vi "HELGA_ECD.vi"() -> ()   [LabVIEW 2017]
panel:
  out "Methoden":T1(array[cluster])
  in  "Tab Control":T2(tab)
  in  "Dateiordner Housekeeping":path=path "C:/Users/Atmos/Desktop/Johnny"
  in  "Dateiname Housekeeping":string
  in  "DateiordnerECD1":path
  in  "DateinameECD1":string
  in  "DateiordnerECD2":path
  in  "DateinameECD2":string
  in  "Modul1/AI sicherer Bereich":dbl[][](array[numeric])=[[0.0, 0.0, 0.0, 0.0, 0.0, 0.0, 0.0, 0.0, 0.0, 0.0, 0.0, 0.0, 0.0, 0.0, 0.0, 0.0, 0.0, 0.0, 0.0, 0.0, 0.0, 0.0, 0.0, 0.0, 0.0, 0.0, 0.0, 0.0, 0.0, 0.0, 0.0, 0.0]]
  in  "Modul1/AIsNamen":string[](array[string])
  in  "Modul1/AI koeff":dbl[][](array[numeric])=[[0.0, 0.0, 0.0, 0.0, 0.0, 0.0, 0.0, 0.0, 0.0, 0.0, 0.0, 0.0, 0.0, 0.0, 0.0, 0.0, 0.0, 0.0, 0.0, 0.0, 0.0, 0.0, 0.0, 0.0, 0.0, 0.0, 0.0, 0.0, 0.0, 0.0, 0.0, 0.0]]
  in  "AIsNamenZurücksetzen":bool
  in  "Modul2/AIsNamen":string[](array[string])
  in  "Modul2/AI koeff":dbl[][](array[numeric])=[[0.0, 0.0, 0.0, 0.0, 0.0, 0.0, 0.0, 0.0, 0.0, 0.0, 0.0, 0.0, 0.0, 0.0, 0.0, 0.0, 0.0, 0.0, 0.0, 0.0, 0.0, 0.0, 0.0, 0.0, 0.0, 0.0, 0.0, 0.0, 0.0, 0.0, 0.0, 0.0]]
  in  "Modul2/AI sicherer Bereich":dbl[][](array[numeric])=[[0.0, 0.0, 0.0, 0.0, 0.0, 0.0, 0.0, 0.0, 0.0, 0.0, 0.0, 0.0, 0.0, 0.0, 0.0, 0.0, 0.0, 0.0, 0.0, 0.0, 0.0, 0.0, 0.0, 0.0, 0.0, 0.0, 0.0, 0.0, 0.0, 0.0, 0.0, 0.0]]
  in  "Modul3/AIsNamen":string[](array[string])
  in  "Modul3/AI koeff":dbl[][](array[numeric])=[[0.0, 0.0, 0.0, 0.0, 0.0, 0.0, 0.0, 0.0, 0.0, 0.0, 0.0, 0.0, 0.0, 0.0, 0.0, 0.0, 0.0, 0.0, 0.0, 0.0, 0.0, 0.0, 0.0, 0.0, 0.0, 0.0, 0.0, 0.0, 0.0, 0.0, 0.0, 0.0]]
  in  "Modul3/AI sicherer Bereich":dbl[][](array[numeric])=[[0.0, 0.0, 0.0, 0.0, 0.0, 0.0, 0.0, 0.0, 0.0, 0.0, 0.0, 0.0, 0.0, 0.0, 0.0, 0.0, 0.0, 0.0, 0.0, 0.0, 0.0, 0.0, 0.0, 0.0, 0.0, 0.0, 0.0, 0.0, 0.0, 0.0, 0.0, 0.0]]
  in  "Traps/MachsKoeff R(U)":dbl[][](array[numeric])=[[0.0, 0.0, 0.0, 0.0, 0.0, 0.0, 0.0, 0.0, 0.0, 0.0, 0.0, 0.0, 0.0, 0.0, 0.0, 0.0, 0.0, 0.0, 0.0, 0.0, 0.0, 0.0, 0.0, 0.0, 0.0, 0.0, 0.0, 0.0, 0.0, 0.0, 0.0, 0.0]]
  out "Schnelle Heizungen":string[](array[string])
  in  "Traps/MachsKoeff T(R)":dbl[][](array[numeric])=[[0.0, 0.0, 0.0, 0.0, 0.0, 0.0, 0.0, 0.0, 0.0, 0.0, 0.0, 0.0, 0.0, 0.0, 0.0, 0.0, 0.0, 0.0, 0.0, 0.0, 0.0, 0.0, 0.0, 0.0, 0.0, 0.0, 0.0, 0.0, 0.0, 0.0, 0.0, 0.0]]
  in  "Traps/Machs sicherer Bereich":dbl[][](array[numeric])=[[0.0, 0.0, 0.0, 0.0, 0.0, 0.0, 0.0, 0.0, 0.0, 0.0, 0.0, 0.0, 0.0, 0.0, 0.0, 0.0, 0.0, 0.0, 0.0, 0.0, 0.0, 0.0, 0.0, 0.0, 0.0, 0.0, 0.0, 0.0, 0.0, 0.0, 0.0, 0.0]]
  in  "LangsameHeizungen":string[](array[string])
  in  "ModuleLH":i32[](array[numeric]) min=1 max=3 step=1
  in  "AIsLH":i32[](array[numeric]) min=0 max=31 step=1
  in  "LHGruppe":bool[](array[boolean])
  in  "DIOsMod0Name":string[](array[string])
  in  "DIOsMod0Nr":i32[](array[numeric]) min=0 max=63 step=1
  in  "DIOsMod1Name":string[](array[string])
  in  "DIOsMod1Nr":i32[](array[numeric]) min=0 max=63 step=1
  in  "DIOsMod2AName":string[](array[string])
  in  "DIOsMod2ANr":i32[](array[numeric]) min=0 max=63 step=1
  in  "DIOsMod2BName":string[](array[string])
  in  "DIOsMod2BNr":i32[](array[numeric]) min=0 max=63 step=1
  out "AnzahlRegler/Modul":i32[](array[numeric])
  in  "Regler für den Probenfluß":i32
  in  "ReglerNameMod0":string[](array[string])
  in  "ReglerNameMod1":string[](array[string])
  in  "ReglerNameMod2A":string[](array[string])
  in  "ReglerNameMod2B":string[](array[string])
  in  "MWabfragenMod0":string[](array[string])=[":060F0401210120", ":06100401210120", ":06110401210120"]
  in  "MWabfragenMod1":string[](array[string])=[":060F0401210120", ":06100401210120", ":06110401210120"]
  in  "MWabfragenMod2A":string[](array[string])=[":060F0401210120", ":06100401210120", ":06110401210120"]
  in  "MWabfragenMod2B":string[](array[string])=[":060F0401210120", ":06100401210120", ":06110401210120"]
  in  "SPvorgebenMod0":string[](array[string])=[":060F020121", ":0610020121", ":0611020121"]
  in  "SPvorgebenMod1":string[](array[string])=[":060F020121", ":0610020121", ":0611020121"]
  in  "SPvorgebenMod2A":string[](array[string])=[":060F020121", ":0610020121", ":0611020121"]
  in  "SPvorgebenMod2B":string[](array[string])=[":060F020121", ":0610020121", ":0611020121"]
  in  "FaktorMod0":dbl[](array[numeric])=[9.375e-05, 9.375e-05, 9.375e-05]
  in  "FaktorMod1":dbl[](array[numeric])=[9.375e-05, 9.375e-05, 9.375e-05]
  in  "FaktorMod2A":dbl[](array[numeric])=[9.375e-05, 9.375e-05, 9.375e-05]
  in  "FaktorMod2B":dbl[](array[numeric])=[9.375e-05, 9.375e-05, 9.375e-05]
  in  "MWAntwortMod0":string[](array[string])=[":060F020121", ":0610020121", ":0611020121"]
  in  "MWAntwortMod1":string[](array[string])=[":060F020121", ":0610020121", ":0611020121"]
  in  "MWAntwortMod2A":string[](array[string])=[":060F020121", ":0610020121", ":0611020121"]
  in  "MWAntwortMod2B":string[](array[string])=[":060F020121", ":0610020121", ":0611020121"]
  in  "ReglerMod0 sicherer Bereich":dbl[][](array[numeric])=[[9.375e-05, 9.375e-05, 9.375e-05]]
  in  "ReglerMod1 sicherer Bereich":dbl[][](array[numeric])=[[9.375e-05, 9.375e-05, 9.375e-05]]
  in  "ReglerMod2A sicherer Bereich":dbl[][](array[numeric])=[[9.375e-05, 9.375e-05, 9.375e-05]]
  in  "ReglerMod2B sicherer Bereich":dbl[][](array[numeric])=[[9.375e-05, 9.375e-05, 9.375e-05]]
  in  "Metavariablen grüner Bereich":dbl[][](array[numeric])=[[0.0, 0.0, 0.0, 0.0, 0.0, 0.0, 0.0, 0.0, 0.0, 0.0, 0.0, 0.0, 0.0, 0.0, 0.0, 0.0, 0.0, 0.0, 0.0, 0.0, 0.0, 0.0, 0.0, 0.0, 0.0, 0.0, 0.0, 0.0, 0.0, 0.0, 0.0, 0.0]]
  in  "Metavariablen":string[](array[string])
  in  "Startmethode":i32=1
  in  "MethodeLöschen":bool
  in  "MethodeDuplizieren":bool
  in  "T_MainMach2":dbl[](array[numeric])
  in  "t_MainMach2":dbl[](array[numeric])
  in  "T_MainMach1":dbl[](array[numeric])
  in  "t_MainMach1":dbl[](array[numeric])
  in  "EinstellungenSpeichern":bool
  out "LangsameHeizungen":string[](array[string])
  in  "AllesSpeichern":bool
  in  "Methodenname":string
  in  "Int.Stop2":dbl
  in  "Int.Start2":dbl
  in  "Int.Stop1":dbl
  in  "Int.Start1":dbl
  in  "ZeitpktMS-2":dbl
  in  "ZeitpktMS-1":dbl
  in  "SPMPV":i32[](array[numeric])
  in  "ZeitpunkteMPV":dbl[](array[numeric])
  in  "Wert2":dbl
  in  "Vergleichsoperator2":dbl(ring) items=["<", "<=", "=", ">=", ">", "=/="]
  in  "AbfragbareVariablen2":dbl(ring) items=["T1-Trap1 [°C]", "T1-Trap2 [°C]", "T1-StirlingKühlkopf [°C]", "T1-PreCol1 [°C]", "T1-PreCol2 [°C]", "T1-MainCol1a [°C]", "T1-MainCol1b [°C]", "T1-MainCol2a [°C]", "T1-MainCol2b [°C]", "T1-Bronkhorst1a [°C]", "T1-Bronkhorst1b [°C]", "T1-Bronkhorst2a [°C]", "T1-Bronkhorst2b [°C]", "T1-2Pos1B [°C]", "T1-Spare9", "T1-2Pos1A [°C]", "T1-Spare10", "T1-TurboPump [°C]", "T1-StirlingPlatine [°C]", "T1-Spare5", "T1-Spare6", "T1-Spare7", "T1-Spare8", "F1-MFM1", "F1-MFM0D [mL]", "P1-HeliumHP [bara]", "P1-HeliumLP [bara]", "P1-PumpVordruck [mbara]", "TurboSpeed", "I1-MS-AC [A]", "I1-Trap1 [A]", "I1-Trap2 [A]", "T2-ECD1a", "T2-ECD1b", "T2-ECD2a", "T2-ECD2b", "T2-Col1a", "T2-Col1b", "T2-Col2a", "T2-Col2b", "T2-Spare1", "T2-Spare2", "T2-Oven_a", "T2-Oven_b", "T2-Spare3", "T2-Spare4", "T2-Spare5", "F2-MFM0", "F2-MFM2A", "F2-MFM2B", "P2-N2O_HP", "P2-N2O_LP", "P2-CO2_HP", "P2-CO2_LP", "AI-Spare1", "FL-MFM1000mL", "AI-Spare3", "AI-Spare4", "StirlingAlarm", "StirlingEmerg.", "AI-Spare7", "AI-Spare8", "AI-Spare9", "FL-MFM30mL", "T0-DC/DC5", "I0-24V_M0", "I0-48V_M1", "I0-24V_M1", "I0-28V_M2", "T0-Spare3", "T0-Spare2", "T0-Spare4", "T0-DC/DC7", "I0-20V_Laptop", "I0-28V_M1", "I0-24V_M2", "I0-12V_Licor", "T0-Spare1", "T0-Drier", "T0-Spare5", "F0-MFM0A [L]", "TL-Licor_a", "P0-Span-HP", "P0-spare1", "P0-Stickstoff-LP", "P0-Helium-LP", "P0-Cal-HP", "P0-P9Tavco[bar]", "F0-MFM0B [L]", "TL-Licor_b", "P0-Span-LP", "P0-spare2", "P0-Stickstoff-HP", "P0-Helium-HP", "P0-Cal-LP", "F0-MFM3", "T-Trap1", "T-Trap2", "T-PreMach1", "T-PreMach2", "T-MainMach1", "T-MainMach2", "PrC0 [bara]", "PrC0-Licor [bara]", "PrC1-Säule1 [bara]", "PrC1-Säule2 [bara]", "MFC1-Sample [ml/min]", "PrC1-BackFlush1 [bara]", "PrC1-BackFlush2 [bara]", "MFC1-Reaktant [l/min]", "MFC2A[ml/min]", "MFC2B[ml/min]", "MFC2C[ul/min]", "PrC2A[bara]", "MFC2D[ml/min]", "MFC2E[ml/min]", "PrC2B[bara]", "Gesamte Zeit", "Methodenzeit", "Zykluszeit Mod0", "Zykluszeit Mod1", "Zykluszeit Mod2A", "Zykluszeit Mod2B", "PositionMPV", "OverflowB", "OverflowA", "StirlingAlarmAlarm!"]
  in  "Dateien fürs MS schicken?":bool
  in  "Zwangsbedingungen":dbl[][](array[numeric])
  out "ZwangsBedingungen":string[][](array[string])
  in  "löschen":bool
  in  "Bedingung Nr. X":i32
  in  "Bedingung übernehmen":bool
  in  "Ausgangswert":dbl
  in  "BedienbareVariablen":dbl(ring) items=["D0-48V_M1", "D0-28V_M1", "D0-Pump2", "DL-LiCalS1H", "D-Spare2", "D-Spare4", "D0-28V_M2", "D0-Pump1", "D0-S01/EV1", "DL-Licor", "D0-EV3", "D0-EV2", "D1-StopMS", "D1-StartMS", "D1-TrapEvac1", "D1-TrapEvac2", "D1-2Pos1A", "D1-2Pos1B", "D1-TurboPump", "D1-PrePump", "D1-VacPump1", "D1-VacPump2", "D1-Stirling", "D1-P_MS", "D1-S1B(7)", "D1-S1A(6)", "D1-S1G", "D1-Fan3", "D1-LüfterMach1", "D1-LüfterMach2", "D1-MS-Power", "D2-SpülflußA", "D2-2Pos2A", "D2-Probe2A", "D2-ECD1HeaterOff", "D2-Fan1", "D2-Fan2", "D2-Spülfluß2B", "D2-2Pos2B", "D2-Probe2B", "D2-ECD2HeaterOff", "Heizen?Trap1", "Heizen?Trap2", "Heizen?PreMach1", "Heizen?PreMach2", "Heizen?MainMach1", "Heizen?MainMach2", "Methodennummer", "STOPP!!!", "H1-Valve1B heizen?", "H1-Bronkhorst1 heizen?", "H1-Bronkhorst2 heizen?", "H1-Valve1A heizen?", "H0-Drier heizen?", "HL-Licor heizen?", "H2-ECD2 heizen?", "H2-Oven heizen?", "H2-Spare1 heizen?", "H2-Col2 heizen?", "H2-Col1 heizen?", "H2-ECD1 heizen?", "PrC0 [bara]", "PrC0-Licor [bara]", "PrC1-Säule1 [bara]", "PrC1-Säule2 [bara]", "MFC1-Sample [ml/min]", "PrC1-BackFlush1 [bara]", "PrC1-BackFlush2 [bara]", "MFC1-Reaktant [l/min]", "MFC2A[ml/min]", "MFC2B[ml/min]", "MFC2C[ul/min]", "PrC2A[bara]", "MFC2D[ml/min]", "MFC2E[ml/min]", "PrC2B[bara]", "PositionMPV", "OverflowB", "OverflowA", "StirlingAlarmAlarm!"]
  in  "Wert1":dbl
  in  "Vergleichsoperator1":dbl(ring) items=["<", "<=", "=", ">=", ">", "=/="]
  in  "AbfragbareVariablen1":dbl(ring) items=["T1-Trap1 [°C]", "T1-Trap2 [°C]", "T1-StirlingKühlkopf [°C]", "T1-PreCol1 [°C]", "T1-PreCol2 [°C]", "T1-MainCol1a [°C]", "T1-MainCol1b [°C]", "T1-MainCol2a [°C]", "T1-MainCol2b [°C]", "T1-Bronkhorst1a [°C]", "T1-Bronkhorst1b [°C]", "T1-Bronkhorst2a [°C]", "T1-Bronkhorst2b [°C]", "T1-2Pos1B [°C]", "T1-Spare9", "T1-2Pos1A [°C]", "T1-Spare10", "T1-TurboPump [°C]", "T1-StirlingPlatine [°C]", "T1-Spare5", "T1-Spare6", "T1-Spare7", "T1-Spare8", "F1-MFM1", "F1-MFM0D [mL]", "P1-HeliumHP [bara]", "P1-HeliumLP [bara]", "P1-PumpVordruck [mbara]", "TurboSpeed", "I1-MS-AC [A]", "I1-Trap1 [A]", "I1-Trap2 [A]", "T2-ECD1a", "T2-ECD1b", "T2-ECD2a", "T2-ECD2b", "T2-Col1a", "T2-Col1b", "T2-Col2a", "T2-Col2b", "T2-Spare1", "T2-Spare2", "T2-Oven_a", "T2-Oven_b", "T2-Spare3", "T2-Spare4", "T2-Spare5", "F2-MFM0", "F2-MFM2A", "F2-MFM2B", "P2-N2O_HP", "P2-N2O_LP", "P2-CO2_HP", "P2-CO2_LP", "AI-Spare1", "FL-MFM1000mL", "AI-Spare3", "AI-Spare4", "StirlingAlarm", "StirlingEmerg.", "AI-Spare7", "AI-Spare8", "AI-Spare9", "FL-MFM30mL", "T0-DC/DC5", "I0-24V_M0", "I0-48V_M1", "I0-24V_M1", "I0-28V_M2", "T0-Spare3", "T0-Spare2", "T0-Spare4", "T0-DC/DC7", "I0-20V_Laptop", "I0-28V_M1", "I0-24V_M2", "I0-12V_Licor", "T0-Spare1", "T0-Drier", "T0-Spare5", "F0-MFM0A [L]", "TL-Licor_a", "P0-Span-HP", "P0-spare1", "P0-Stickstoff-LP", "P0-Helium-LP", "P0-Cal-HP", "P0-P9Tavco[bar]", "F0-MFM0B [L]", "TL-Licor_b", "P0-Span-LP", "P0-spare2", "P0-Stickstoff-HP", "P0-Helium-HP", "P0-Cal-LP", "F0-MFM3", "T-Trap1", "T-Trap2", "T-PreMach1", "T-PreMach2", "T-MainMach1", "T-MainMach2", "PrC0 [bara]", "PrC0-Licor [bara]", "PrC1-Säule1 [bara]", "PrC1-Säule2 [bara]", "MFC1-Sample [ml/min]", "PrC1-BackFlush1 [bara]", "PrC1-BackFlush2 [bara]", "MFC1-Reaktant [l/min]", "MFC2A[ml/min]", "MFC2B[ml/min]", "MFC2C[ul/min]", "PrC2A[bara]", "MFC2D[ml/min]", "MFC2E[ml/min]", "PrC2B[bara]", "Gesamte Zeit", "Methodenzeit", "Zykluszeit Mod0", "Zykluszeit Mod1", "Zykluszeit Mod2A", "Zykluszeit Mod2B", "PositionMPV", "OverflowB", "OverflowA", "StirlingAlarmAlarm!"]
  in  "Methode Nummer":i32
  in  "MethodeLaden":bool
  in  "EditorBeenden":bool
  in  "PIDs für \"träge\" Heizungen":T3(array[cluster])
  in  "T_PreMach2":dbl[](array[numeric])
  in  "t_PreMach2":dbl[](array[numeric])
  in  "T_PreMach1":dbl[](array[numeric])
  in  "t_PreMach1":dbl[](array[numeric])
  in  "SHSetpoints":dbl[][](array[numeric])
  in  "ZeitpktFPGAFixp":dbl[](array[numeric])
  in  "FPGAPID":T4(array[cluster])
  in  "ZeitpktFPGAPID":dbl[](array[numeric])
  in  "FPGABoolesch":bool[][](array[boolean])
  in  "ZPktFPGABoolesch":dbl[](array[numeric])
  in  "LHHeizen?":bool[](array[boolean])
  in  "LHSetpoints":dbl[](array[numeric])
  out "HorstMod1Name":string[](array[string])
  out "HorstMod2AName":string[](array[string])
  out "HorstMod2BName":string[](array[string])
  in  "HorstSPMod1":dbl[][](array[numeric])
  in  "HorstSPMod2A":dbl[][](array[numeric])
  in  "HorstSPMod2B":dbl[][](array[numeric])
  in  "Mod1HorstZeitpkt":dbl[](array[numeric])
  in  "Mod2AHorstZeitpkt":dbl[](array[numeric])
  in  "Mod2BHorstZeitpkt":dbl[](array[numeric])
  in  "HorstSPMod0":dbl[][](array[numeric])
  out "HorstMod0Name":string[](array[string])
  in  "Mod0HorstZeitpkt":dbl[](array[numeric])
  in  "DIOsSPMod2B":bool[][](array[boolean])
  in  "DIOsSPMod2A":bool[][](array[boolean])
  in  "DIOsSPMod1":bool[][](array[boolean])
  in  "ZeitpktDIOsMod2B":dbl[](array[numeric])
  in  "ZeitpktDIOsMod2A":dbl[](array[numeric])
  in  "ZeitpktDIOsMod1":dbl[](array[numeric])
  out "DIOsMod2BName":string[](array[string])
  out "DIOsMod2AName":string[](array[string])
  out "DIOsMod1Name":string[](array[string])
  out "DIOsMod0Name":string[](array[string])
  in  "DIOsSPMod0":bool[][](array[boolean])
  in  "ZeitpktDIOsMod0":dbl[](array[numeric])
  in  "MethodeSpeichern":bool
  in  "EinstellungenFertig":bool
  in  "Zykluslängen [s]":dbl[](array[numeric])
  # "Trap1          Trap2      PreMach1  PreMach2 MainMach1 MainMach2\n       heizen         heizen        heizen         heizen         heizen         heizen"
  # "Trap1"
  # "Trap2"
  # "PreMach1"
  # "PreMach2"
  # "MainMach1"
  # "MainMach2"
  # "Sososo... alle Einstellungen vorgenommen? Wirklich alle? Sicher? Bereit, mit den Methoden fortzufahren? Na super, dann trau Dich und drück den Knopf!"
  # "Es können beliebig viele Methoden definiert werden; die gewünschte Nummer auswählen und die entsprechende Methode laden, dann nach Belieben dran rumfummeln und anschließend, wenns beliebt, die vorgenommenen Änderungen an der Methode übernehmen (das bedeutet NICHT, daß die Änderungen in einer Datei abgelegt werden, dafür gibts nen extra Knopp);\n\"Editor beenden\" dürfte klar sein. Und Tschüß!"
  # ":::Tom \"Awesome\"  Burner Jr.:::"
  # "Sollen die Daten vom MS abgefragt werden? Wenn ja, zu welchen Zeitpunkten (im Zyklus1)?"
  # "Schnelle Heizungen..."
  # "Die eingegebenen Punkte im (t-T)-Raum werden durch lineare Funktionen verbunden, jeweils definiert von Punkt zu Punkt."
  # "Stellung des Multipositionsventils; die Zeitpunkte beziehen sich auf den Zyklus von Modul0.\nDie Stellungen bezeichnen: \n1. Cal - 2. Span - 3. ? - 4. ? - \n5. Plank - 6. Air - 7. ?"
  # "Innerhalb welcher Zeitfenster (Modul1) soll der Probenfluß integriert werden?"
  # "Der Gipfel der Flexibilität: die Zwangsbedingungen!\nBitte boolesche Werte als 0/1 eingeben"
  # "Mod0\n\nMod1\n\nMod2A\n\nMod2B"
  # "UND"
  # "TSetpTrap1                TSetpTrap2"
  # "Dran denken: die Daten werden auf dem CRIO abgelegt, nicht auf dem ITX oder dem Notebook; Dateinamen bitte ohne Pfad und .tdms eingeben!"
  # "Die Analogeingänge sind entsprechend der AI-Module des CRIO angeordnet (3x32); es wird eine quadratische Kennlinie angenommen, also: y=a0+a1*x+a2*x^2;\ndie drei Koeffizienten werden in dieser Reihenfolge eingegeben (v.l.n.r.): a0, a1, a2. Die Alarmgrenzen werden folgendermaßen eingegeben: linke Spalte für untere Grenze, rechte Spalte für obere Grenze des sicheren Bereichs."
  # "Die Analogeingänge sind entsprechend der AI-Module des CRIO angeordnet (3x32); es wird eine quadratische Kennlinie angenommen, also: y=a0+a1*x+a2*x^2;\ndie drei Koeffizienten werden in dieser Reihenfolge eingegeben (v.l.n.r.): a0, a1, a2. Die Alarmgrenzen werden folgendermaßen eingegeben: linke Spalte für untere Grenze, rechte Spalte für obere Grenze des sicheren Bereichs."
  # "Die Analogeingänge sind entsprechend der AI-Module des CRIO angeordnet (3x32); es wird eine quadratische Kennlinie angenommen, also: y=a0+a1*x+a2*x^2;\ndie drei Koeffizienten werden in dieser Reihenfolge eingegeben (v.l.n.r.): a0, a1, a2. Die Alarmgrenzen werden folgendermaßen eingegeben: linke Spalte für untere Grenze, rechte Spalte für obere Grenze des sicheren Bereichs."
  # "Vorsicht!!! Wer hier nicht ganz genau weiß, was er tut, läßt bitte die Finger davon!\nDie Heizungen werden über den FPGA gesteuert, d.h. wenn man die Anzahl oder die Anschlüsse der Heizungen ändert, muß das FPGA-Programm entsprechend angepaßt werden.\nModuleLH bezieht sich auf die drei AI-Module des CRIO (1,2,3) und AIsLH auf den Anschluß im jeweiligen Modul."
  # "Die digitalen Ein-/Ausgänge werden modulweise aufgelistet (0, 1, 2A, 2B) und benannt; die zugehörigen Anschlüsse werden folgendermaßen durchgezählt: \nDIO 0...31 von Modul5 entspricht hier 0...31; DIO 0...31 von Modul6 entspricht hier 32+(0...31)=32...63."
  # "Die Bronkhorst-Regler werden modulweise zusammengefasst an den CRIO angeschlossen, Mod0 an Port0, Mod1 an Port1, Mod2A&2B an Port2;\ndie Strings für die Steuerung und Abfrage der Regler ergeben sich aus dem bronkhorstschen Handbuch; der Faktor berechnet sich durch \"Vollausschlag des Reglers (in der gewünschten Einheit, z.B. Bar)\"/32000;\n'Regler für den Probenfluß' meint die Nummer des entsprechenden Reglers in der Liste aller Regler, wobei der erste die Nummer 0 trägt."
  # "Wer will noch mehr, wer hat noch nichts? An dieser Stelle können weitere Variablen definiert werden, mit deren Hilfe die Zwangsbedingungen erst ihre volle Pracht und Mächtigkeit entfalten. Alle Variablen sind numerische Größen und haben damit beliebig viele Zustände. Beim Programmstart werden sie mit Null initialisiert.\nHöchschte Vorsicht ist beim Umbenennen oder gar Löschen von Variablen geboten, weil sich das fatal auf bestehende Zwangsbedingungen auswirken kann. Am besten immer nur neue Variablen hinzufügen, das garantiert sicheren Spaß ohne Spätfolgen."
  # "Im weiteren können beliebig viele Methoden definiert werden; mit welcher davon soll das Programm starten? Die erste Methode trägt die Nummer 0."
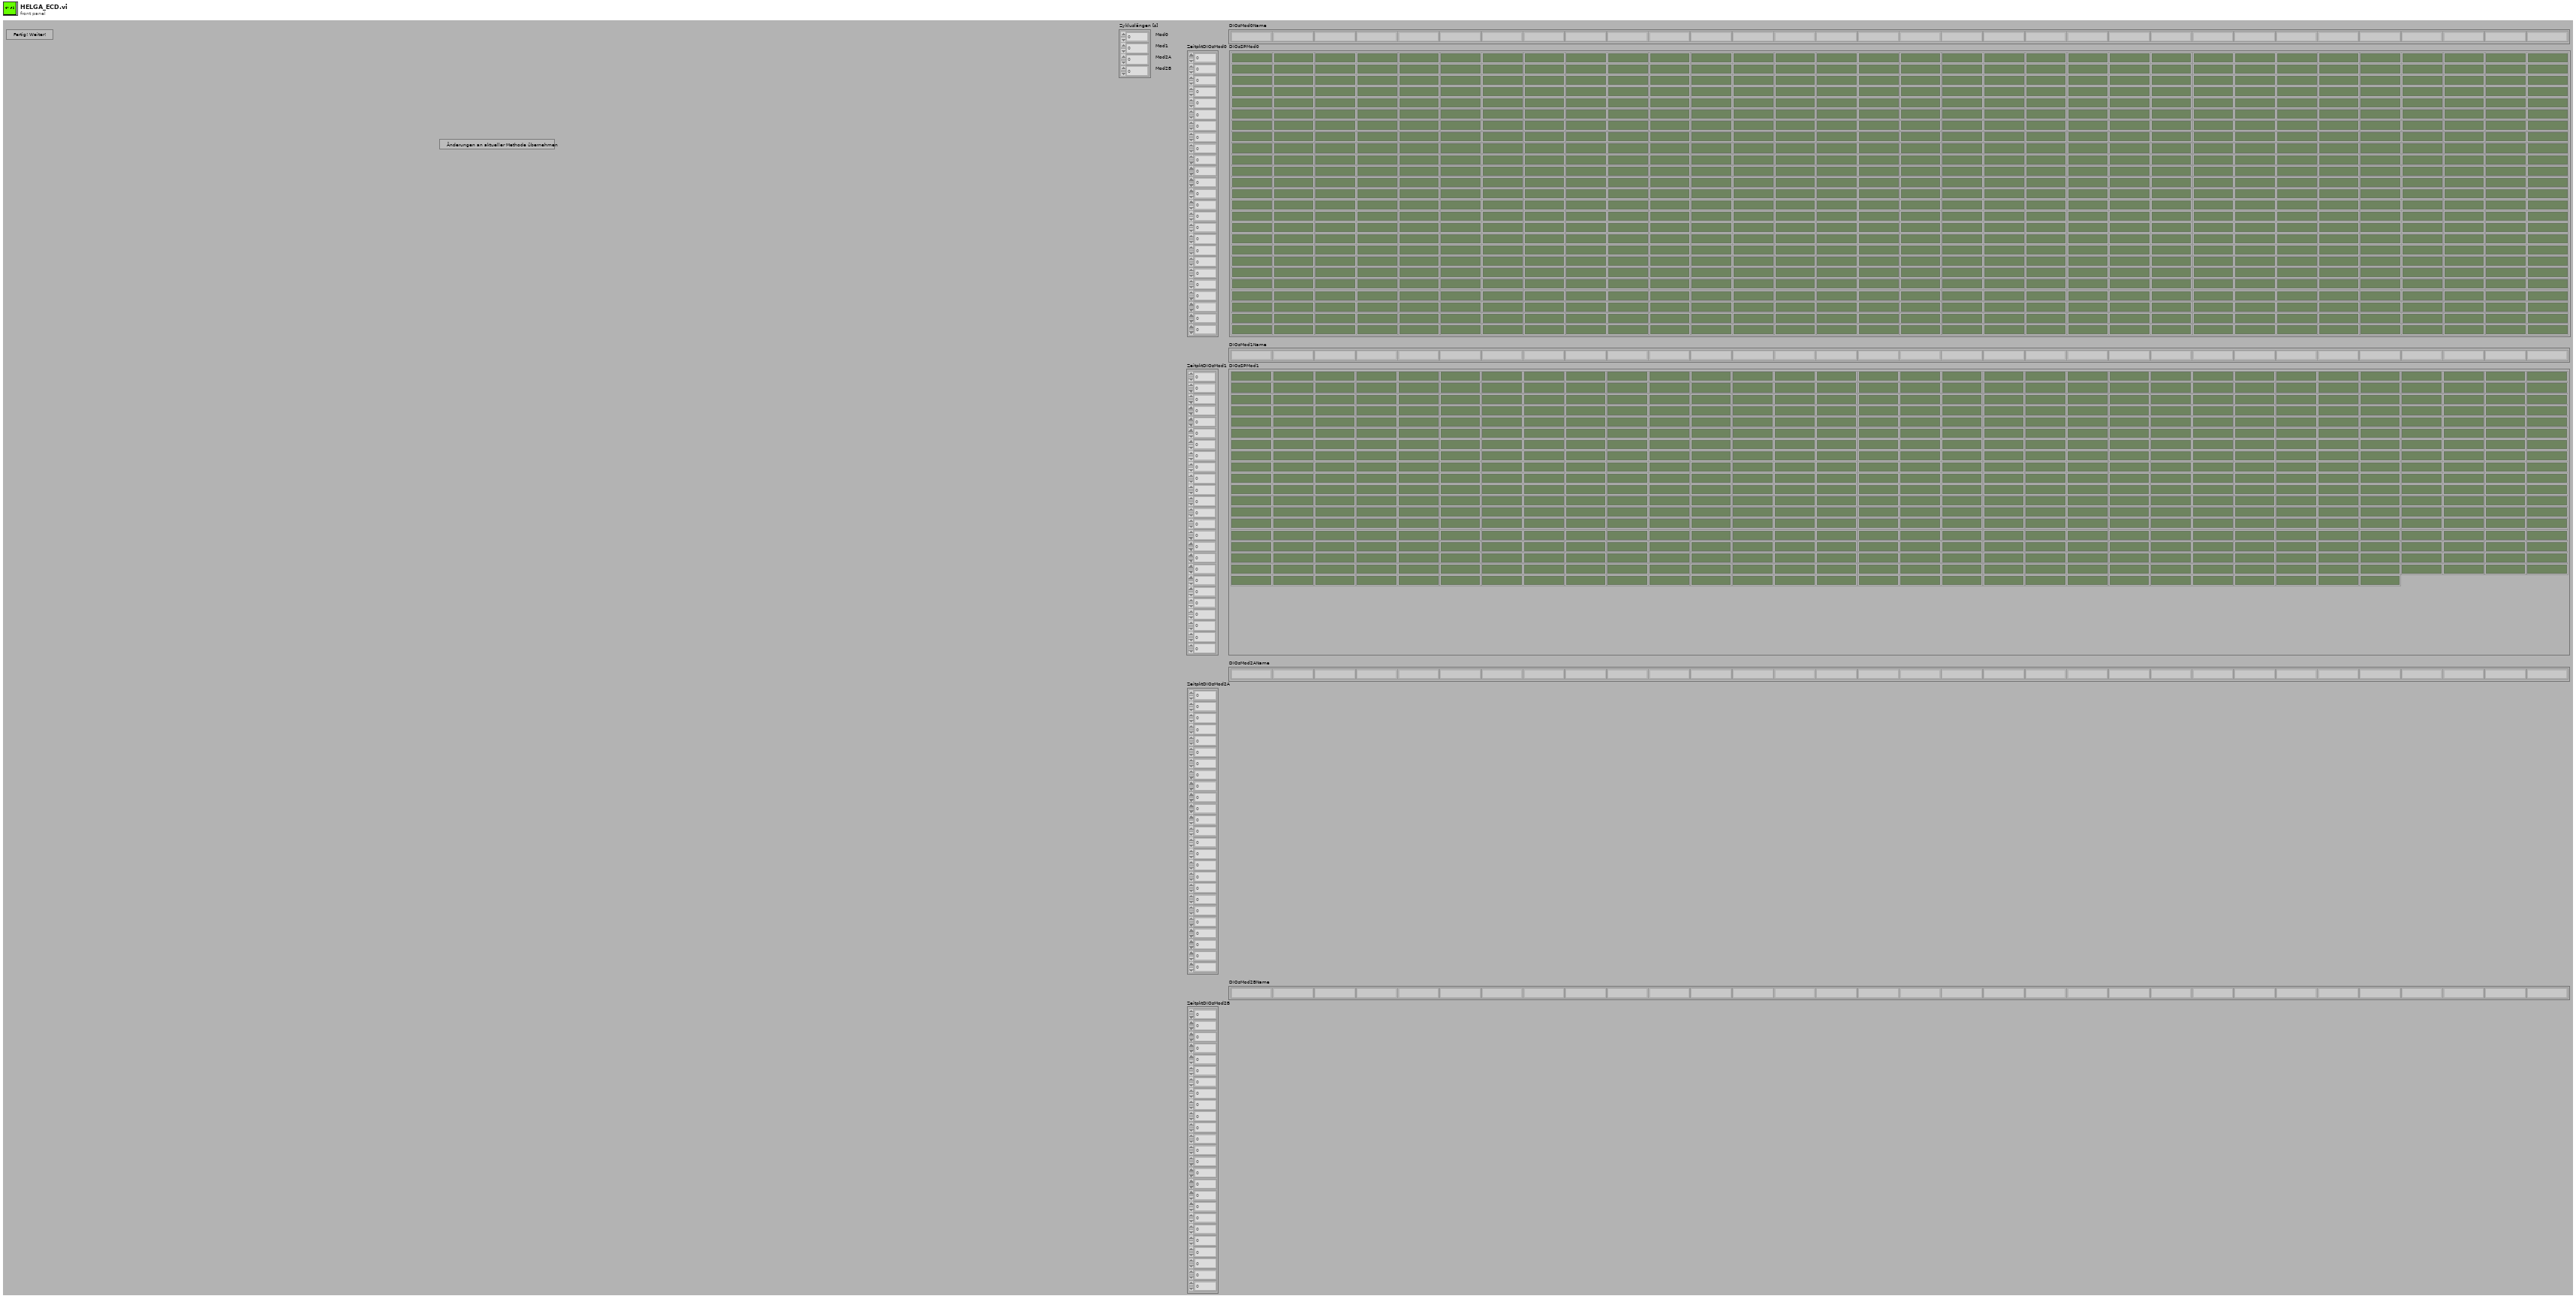
[diagram p1: front panel]
types:
  T1 = cluster{"Zykluslängen [s]":dbl[], "ZeitpktDIOsMod0":dbl[], "ZeitpktDIOsMod1":dbl[], "ZeitpktDIOsMod2A":dbl[], "ZeitpktDIOsMod2B":dbl[], "DIOsSPMod0":bool[][], "DIOsSPMod1":bool[][], "DIOsSPMod2A":bool[][], "DIOsSPMod2B":bool[][], "Mod0HorstZeitpkt":dbl[], "Mod1HorstZeitpkt":dbl[], "Mod2AHorstZeitpkt":dbl[], "Mod2BHorstZeitpkt":dbl[], "HorstSPMod0":dbl[][], "HorstSPMod1":dbl[][], "HorstSPMod2A":dbl[][], "HorstSPMod2B":dbl[][], "LHSetpoints":dbl[], "LHHeizen?":bool[], "ZPktFPGABoolesch":dbl[], "FPGABoolesch":bool[][], "ZeitpktFPGAPID":dbl[], "FPGAPID":cluster{"d0":fxp<+/-,18,18>, "d1":fxp<+/-,21,21>}[][], "ZeitpktFPGAFixp":dbl[], "SHSetpoints":dbl[][], "t_PreMach1":dbl[], "T_PreMach1":dbl[], "t_PreMach2":dbl[], "T_PreMach2":dbl[], "PIDs für \"träge\" Heizungen":cluster{"proportional gain (Kc)":dbl, "integral time (Ti, min)":dbl, "derivative time (Td, min)":dbl}[], "Zwangsbedingungen":dbl[][], "Dateien fürs MS schicken?":bool, "ZeitpunkteMPV":dbl[], "SPMPV":i32[], "ZeitpktMS-1":dbl, "ZeitpktMS-2":dbl, "Int.Start1":dbl, "Int.Stop1":dbl, "Int.Start2":dbl, "Int.Stop2":dbl, "Methodenname":string, "t_MainMach1":dbl[], "T_MainMach1":dbl[], "t_MainMach2":dbl[], "T_MainMach2":dbl[]}[]
  T2 = enum32{"Dateinamen", "Modul1/AIs", "Modul2/AIs", "Modul3/AIs", "schnelle Heizungen", "langsame Heizungen", "DIOs", "Horst-Regler", "Metavariablen", "Startmethode"}
  T3 = cluster{"proportional gain":dbl, "integral time":dbl, "derivative time":dbl}[]
  T4 = cluster{"d0":fxp<+/-,18,18>, "d1":fxp<+/-,21,21>}[][]
  T5 = cluster{"DIOsMod0Nr":i32[], "DIOsMod1Nr":i32[], "DIOsMod2ANr":i32[], "DIOsMod2BNr":i32[], "AIsLH":i32[], "AnzahlRegler/Modul":i32[], "Regler für den Probenfluß":i32, "SPvorgebenMod0":string[], "SPvorgebenMod1":string[], "SPvorgebenMod2A":string[], "SPvorgebenMod2B":string[], "MWAntwortMod0":string[], "MWAntwortMod1":string[], "MWAntwortMod2A":string[], "MWAntwortMod2B":string[], "FaktorMod0":dbl[], "FaktorMod1":dbl[], "FaktorMod2A":dbl[], "FaktorMod2B":dbl[], "MWabfragenMod0":string[], "MWabfragenMod1":string[], "MWabfragenMod2A":string[], "MWabfragenMod2B":string[], "Modul1/AI koeff":dbl[][], "Modul2/AI koeff":dbl[][], "Modul3/AI koeff":dbl[][], "Traps/MachsKoeff T(R)":dbl[][], "Modul1/AIsNamen":string[], "Modul2/AIsNamen":string[], "Modul3/AIsNamen":string[], "DIOsMod0Name":string[], "DIOsMod1Name":string[], "DIOsMod2AName":string[], "DIOsMod2BName":string[], "ReglerNameMod0":string[], "ReglerNameMod1":string[], "ReglerNameMod2A":string[], "ReglerNameMod2B":string[], "Startmethode":i32, "Dateiordner Housekeeping":path, "Dateiname Housekeeping":string, "DateiordnerECD1":path, "DateinameECD1":string, "DateiordnerECD2":path, "DateinameECD2":string, "LangsameHeizungen":string[], "ModuleLH":i32[], "Metavariablen":string[], "Modul1/AI sicherer Bereich":dbl[][], "Modul2/AI sicherer Bereich":dbl[][], "Modul3/AI sicherer Bereich":dbl[][], "Traps/Machs sicherer Bereich":dbl[][], "ReglerMod0 sicherer Bereich":dbl[][], "ReglerMod1 sicherer Bereich":dbl[][], "ReglerMod2A sicherer Bereich":dbl[][], "ReglerMod2B sicherer Bereich":dbl[][], "Metavariablen grüner Bereich":dbl[][], "Traps/MachsKoeff R(U)":dbl[][], "LHGruppe":bool[]}
  T6 = enum16{"open", "replace", "create", "open or create", "replace or create", "replace or create with confirmation"}
  T7 = cluster{"Zykluslängen [s]":dbl[], "ZeitpktDIOsMod0":dbl[], "ZeitpktDIOsMod1":dbl[], "ZeitpktDIOsMod2A":dbl[], "ZeitpktDIOsMod2B":dbl[], "DIOsSPMod0":bool[][], "DIOsSPMod1":bool[][], "DIOsSPMod2A":bool[][], "DIOsSPMod2B":bool[][], "Mod0HorstZeitpkt":dbl[], "Mod1HorstZeitpkt":dbl[], "Mod2AHorstZeitpkt":dbl[], "Mod2BHorstZeitpkt":dbl[], "HorstSPMod0":dbl[][], "HorstSPMod1":dbl[][], "HorstSPMod2A":dbl[][], "HorstSPMod2B":dbl[][], "LHSetpoints":dbl[], "LHHeizen?":bool[], "ZPktFPGABoolesch":dbl[], "FPGABoolesch":bool[][], "ZeitpktFPGAPID":dbl[], "FPGAPID":cluster{"d0":fxp<+/-,18,18>, "d1":fxp<+/-,21,21>}[][], "ZeitpktFPGAFixp":dbl[], "SHSetpoints":dbl[][], "t_PreMach1":dbl[], "T_PreMach1":dbl[], "t_PreMach2":dbl[], "T_PreMach2":dbl[], "PIDs für \"träge\" Heizungen":cluster{"proportional gain (Kc)":dbl, "integral time (Ti, min)":dbl, "derivative time (Td, min)":dbl}[], "Zwangsbedingungen":dbl[][], "Dateien fürs MS schicken?":bool, "ZeitpunkteMPV":dbl[], "SPMPV":i32[], "ZeitpktMS-1":dbl, "ZeitpktMS-2":dbl, "Int.Start1":dbl, "Int.Stop1":dbl, "Int.Start2":dbl, "Int.Stop2":dbl, "Methodenname":string, "t_MainMach1":dbl[], "T_MainMach1":dbl[], "t_MainMach2":dbl[], "T_MainMach2":dbl[]}
  T8 = cluster{"proportional gain (Kc)":dbl, "integral time (Ti, min)":dbl, "derivative time (Td, min)":dbl}[]
  T9 = cluster{"Zykluslängen [s]":dbl[], "ZeitpktDIOsMod0":dbl[], "ZeitpktDIOsMod1":dbl[], "ZeitpktDIOsMod2A":dbl[], "ZeitpktDIOsMod2B":dbl[], "DIOsSPMod0":bool[][], "DIOsSPMod1":bool[][], "DIOsSPMod2A":bool[][], "DIOsSPMod2B":bool[][], "Mod0HorstZeitpkt":dbl[], "Mod1HorstZeitpkt":dbl[], "Mod2AHorstZeitpkt":dbl[], "Mod2BHorstZeitpkt":dbl[], "HorstSPMod0":dbl[][], "HorstSPMod1":dbl[][], "HorstSPMod2A":dbl[][], "HorstSPMod2B":dbl[][], "LHSetpoints":dbl[], "LHHeizen?":bool[], "ZPktFPGABoolesch":dbl[], "FPGABoolesch":bool[][], "ZeitpktFPGAPID":dbl[], "FPGAPID":cluster{"d0":fxp<+/-,18,18>, "d1":fxp<+/-,21,21>}[][], "ZeitpktFPGAFixp":dbl[], "SHSetpoints":dbl[][], "t_PreMach1":dbl[], "T_PreMach1":dbl[], "t_PreMach2":dbl[], "T_PreMach2":dbl[], "PIDs für \"träge\" Heizungen":cluster{"proportional gain":dbl, "integral time":dbl, "derivative time":dbl}[], "Zwangsbedingungen":dbl[][], "Dateien fürs MS schicken?":bool, "ZeitpunkteMPV":dbl[], "SPMPV":i32[], "ZeitpktMS-1":dbl, "ZeitpktMS-2":dbl, "Int.Start1":dbl, "Int.Stop1":dbl, "Int.Start2":dbl, "Int.Stop2":dbl, "Methodenname":string, "t_MainMach1":dbl[], "T_MainMach1":dbl[], "t_MainMach2":dbl[], "T_MainMach2":dbl[]}
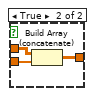
[diagram p9: hidden frame]
diagram:
  n1 = Open/Create/Replace File(file path (use dialog)=path "c:/einstellungen.pery" ("Dateipfad Einstellungen")) -> (refnum out=w19:refnum<file>, error out=w20:errorcluster)  [unwired: 5 in, 1 out]
  n2 = Read from Binary File(5:T5 {"DIOsMod0Nr"=[], "DIOsMod1Nr"=[], "DIOsMod2ANr"=[], "DIOsMod2BNr"=[], "AIsLH"=[], "AnzahlRegler/Modul"=[], "Regler für den Probenfluß"=0, "SPvorgebenMod0"=[], "SPvorgebenMod1"=[], "SPvorgebenMod2A"=[], "SPvorgebenMod2B"=[], "MWAntwortMod0"=[], "MWAntwortMod1"=[], "MWAntwortMod2A"=[], "MWAntwortMod2B"=[], "FaktorMod0"=[], "FaktorMod1"=[], "FaktorMod2A"=[], "FaktorMod2B"=[], "MWabfragenMod0"=[], "MWabfragenMod1"=[], "MWabfragenMod2A"=[], "MWabfragenMod2B"=[], "Modul1/AI koeff"=[], "Modul2/AI koeff"=[], "Modul3/AI koeff"=[], "Traps/MachsKoeff T(R)"=[], "Modul1/AIsNamen"=[], "Modul2/AIsNamen"=[], "Modul3/AIsNamen"=[], "DIOsMod0Name"=[], "DIOsMod1Name"=[], "DIOsMod2AName"=[], "DIOsMod2BName"=[], "ReglerNameMod0"=[], "ReglerNameMod1"=[], "ReglerNameMod2A"=[], "ReglerNameMod2B"=[], "Startmethode"=0, "Dateiordner Housekeeping"=path "", "Dateiname Housekeeping"="", "DateiordnerECD1"=path "", "DateinameECD1"="", "DateiordnerECD2"=path "", "DateinameECD2"="", "LangsameHeizungen"=[], "ModuleLH"=[], "Metavariablen"=[], "Modul1/AI sicherer Bereich"=[], "Modul2/AI sicherer Bereich"=[], "Modul3/AI sicherer Bereich"=[], "Traps/Machs sicherer Bereich"=[], "ReglerMod0 sicherer Bereich"=[], "ReglerMod1 sicherer Bereich"=[], "ReglerMod2A sicherer Bereich"=[], "ReglerMod2B sicherer Bereich"=[], "Metavariablen grüner Bereich"=[], "Traps/MachsKoeff R(U)"=[], "LHGruppe"=[]} ("output cluster"), 8:w20, 11:w19) -> (0:w17:errorcluster, 2:w5:T5, 3:w18:refnum<file>)  [unwired: 3 in, 1 out]
  n3 = Close File(refnum=w18, error in=w17) -> (error out=w16:errorcluster)  [unwired: 1 out]
  n4 = flat-sequence {
    tunnel: w5 -> [w97]
    tunnel: [w50] -> w8
    tunnel: [w119] -> w36
    tunnel: [w118] -> w35
    tunnel: [w117] -> w34
    tunnel: [w116] -> w33
    tunnel: [w115] -> w32
    tunnel: [w114] -> w31
    tunnel: [w113] -> w30
    tunnel: [w112] -> w29
    tunnel: [w111] -> w28
    tunnel: [w106] -> w27
    tunnel: [w105] -> w26
    tunnel: [w104] -> w25
    tunnel: [w103] -> w24
    tunnel: [w102] -> w23
    tunnel: [w101] -> w22
    tunnel: [w100] -> w9
    tunnel: w8 -> [w100]
    tunnel: [w99] -> w7
    tunnel: [w98] -> w6
    tunnel: w36 -> [w238]
    tunnel: w35 -> [w237]
    tunnel: w34 -> [w236]
    tunnel: w33 -> [w235]
    tunnel: w32 -> [w234]
    tunnel: w31 -> [w233]
    tunnel: w30 -> [w231]
    tunnel: w29 -> [w232]
    tunnel: w28 -> [w230]
    tunnel: w27 -> [w217]
    tunnel: w26 -> [w228]
    tunnel: w25 -> [w227]
    tunnel: w24 -> [w226]
    tunnel: w23 -> [w225]
    tunnel: w22 -> [w220]
    tunnel: w3 -> [w219]
    tunnel: w9 -> [w216]
    tunnel: w7 -> [w214]
    tunnel: w6 -> [w212]
    tunnel: w4 -> [w208]
    frame #0 {
      n5 = Unbundle(w97) -> ("DIOsMod0Nr"=w96:i32[], "DIOsMod1Nr"=w95:i32[], "DIOsMod2ANr"=w94:i32[], "DIOsMod2BNr"=w93:i32[], "AIsLH"=w92:i32[], "AnzahlRegler/Modul"=w91:i32[], "Regler für den Probenfluß"=w90:i32, "SPvorgebenMod0"=w89:string[], "SPvorgebenMod1"=w88:string[], "SPvorgebenMod2A"=w87:string[], "SPvorgebenMod2B"=w86:string[], "MWAntwortMod0"=w85:string[], "MWAntwortMod1"=w84:string[], "MWAntwortMod2A"=w83:string[], "MWAntwortMod2B"=w82:string[], "FaktorMod0"=w81:dbl[], "FaktorMod1"=w80:dbl[], "FaktorMod2A"=w79:dbl[], "FaktorMod2B"=w78:dbl[], "MWabfragenMod0"=w77:string[], "MWabfragenMod1"=w76:string[], "MWabfragenMod2A"=w75:string[], "MWabfragenMod2B"=w74:string[], "Modul1/AI koeff"=w73:dbl[][], "Modul2/AI koeff"=w72:dbl[][], "Modul3/AI koeff"=w71:dbl[][], "Traps/MachsKoeff T(R)"=w70:dbl[][], "Modul1/AIsNamen"=w69:string[], "Modul2/AIsNamen"=w68:string[], "Modul3/AIsNamen"=w67:string[], "DIOsMod0Name"=w66:string[], "DIOsMod1Name"=w65:string[], "DIOsMod2AName"=w64:string[], "DIOsMod2BName"=w63:string[], "ReglerNameMod0"=w62:string[], "ReglerNameMod1"=w61:string[], "ReglerNameMod2A"=w60:string[], "ReglerNameMod2B"=w59:string[], "Startmethode"=w58:i32, "Dateiordner Housekeeping"=w48:path, "Dateiname Housekeeping"=w57:string, "DateiordnerECD1"=w56:path, "DateinameECD1"=w55:string, "DateiordnerECD2"=w54:path, "DateinameECD2"=w53:string, "LangsameHeizungen"=w50:string[], "ModuleLH"=w51:i32[], "Metavariablen"=w49:string[], "Modul1/AI sicherer Bereich"=w47:dbl[][], "Modul2/AI sicherer Bereich"=w46:dbl[][], "Modul3/AI sicherer Bereich"=w45:dbl[][], "Traps/Machs sicherer Bereich"=w44:dbl[][], "ReglerMod0 sicherer Bereich"=w43:dbl[][], "ReglerMod1 sicherer Bereich"=w42:dbl[][], "ReglerMod2A sicherer Bereich"=w41:dbl[][], "ReglerMod2B sicherer Bereich"=w40:dbl[][], "Metavariablen grüner Bereich"=w39:dbl[][], "Traps/MachsKoeff R(U)"=w38:dbl[][], "LHGruppe"=w37:bool[])
      n6 = property on="Modul1/AI sicherer Bereich" class="Arr (strikt)"("Value"=w47) -> ()  [unwired: 2 in, 2 out]
      n7 = property on="Modul3/AI sicherer Bereich" class="Arr (strikt)"("Value"=w45) -> ()  [unwired: 2 in, 2 out]
      n8 = property on="ReglerMod0 sicherer Bereich" class="Arr (strikt)"("Value"=w43) -> ()  [unwired: 2 in, 2 out]
      n9 = property on="ReglerMod1 sicherer Bereich" class="Arr (strikt)"("Value"=w42) -> ()  [unwired: 2 in, 2 out]
      n10 = property on="Modul2/AI sicherer Bereich" class="Arr (strikt)"("Value"=w46) -> ()  [unwired: 2 in, 2 out]
      n11 = property on="Traps/Machs sicherer Bereich" class="Arr (strikt)"("Value"=w44) -> ()  [unwired: 2 in, 2 out]
      n12 = property on="ReglerMod2A sicherer Bereich" class="Arr (strikt)"("Value"=w41) -> ()  [unwired: 2 in, 2 out]
      n13 = property on="ReglerMod2B sicherer Bereich" class="Arr (strikt)"("Value"=w40) -> ()  [unwired: 2 in, 2 out]
      n14 = property on="Metavariablen grüner Bereich" class="Arr (strikt)"("Value"=w39) -> ()  [unwired: 2 in, 2 out]
      n15 = property on="LHGruppe" class="Arr (strikt)"("Value"=w37) -> ()  [unwired: 2 in, 2 out]
      n16 = property on="Traps/MachsKoeff R(U)" class="Arr (strikt)"("Value"=w38) -> ()  [unwired: 2 in, 2 out]
      n17 = invoke on="MethodeLöschen" class="Bool (strict)" method="Std wiederherstellen"() -> ()  [unwired: 3 in, 3 out]
      n18 = property on="ModuleLH" class="Arr (strikt)"("Value"=w51) -> ()  [unwired: 2 in, 2 out]
      n19 = property on="AIsLH" class="Arr (strikt)"("Value"=w92) -> ()  [unwired: 2 in, 2 out]
      n20 = property on="Dateiname Housekeeping" class="Str"("Value"=w57) -> ()  [unwired: 2 in, 2 out]
      n21 = property on="DIOsMod0Nr" class="Arr (strikt)"("Value"=w96) -> ()  [unwired: 2 in, 2 out]
      n22 = property on="DateiordnerECD1" class="Pfad"("Value"=w56) -> ()  [unwired: 2 in, 2 out]
      n23 = property on="DIOsMod1Nr" class="Arr (strikt)"("Value"=w95) -> ()  [unwired: 2 in, 2 out]
      n24 = property on="DateinameECD1" class="Str"("Value"=w55) -> ()  [unwired: 2 in, 2 out]
      n25 = property on="DateiordnerECD2" class="Pfad"("Value"=w54) -> ()  [unwired: 2 in, 2 out]
      n26 = property on="DateinameECD2" class="Str"("Value"=w53) -> ()  [unwired: 2 in, 2 out]
      n27 = property on="DIOsMod2ANr" class="Arr (strikt)"("Value"=w94) -> ()  [unwired: 2 in, 2 out]
      n28 = property on="LangsameHeizungen" class="Arr (strikt)"("Value"=w50) -> ()  [unwired: 2 in, 2 out]
      n29 = property on="Metavariablen" class="Arr (strikt)"("Value"=w49) -> ()  [unwired: 2 in, 2 out]
      n30 = property on="DIOsMod2BNr" class="Arr (strikt)"("Value"=w93) -> ()  [unwired: 2 in, 2 out]
      n31 = property on="AnzahlRegler/Modul" class="Arr (strikt)"("Value"=w91) -> ()  [unwired: 2 in, 2 out]
      n32 = property on="Regler für den Probenfluß" class="DigWert (strikt)"("Value"=w90) -> ()  [unwired: 2 in, 2 out]
      n33 = property on="SPvorgebenMod0" class="Arr (strikt)"("Value"=w89) -> ()  [unwired: 2 in, 2 out]
      n34 = property on="ReglerNameMod2B" class="Arr (strikt)"("Value"=w59) -> ()  [unwired: 2 in, 2 out]
      n35 = property on="Startmethode" class="DigWert (strikt)"("Value"=w58) -> ()  [unwired: 2 in, 2 out]
      n36 = property on="Dateiordner Housekeeping" class="Pfad"("Value"=w48) -> ()  [unwired: 2 in, 2 out]
      n37 = property on="SPvorgebenMod1" class="Arr (strikt)"("Value"=w88) -> ()  [unwired: 2 in, 2 out]
      n38 = property on="SPvorgebenMod2A" class="Arr (strikt)"("Value"=w87) -> ()  [unwired: 2 in, 2 out]
      n39 = property on="SPvorgebenMod2B" class="Arr (strikt)"("Value"=w86) -> ()  [unwired: 2 in, 2 out]
      n40 = property on="MWAntwortMod0" class="Arr (strikt)"("Value"=w85) -> ()  [unwired: 2 in, 2 out]
      n41 = property on="MWAntwortMod1" class="Arr (strikt)"("Value"=w84) -> ()  [unwired: 2 in, 2 out]
      n42 = property on="MWAntwortMod2A" class="Arr (strikt)"("Value"=w83) -> ()  [unwired: 2 in, 2 out]
      n43 = property on="MWAntwortMod2B" class="Arr (strikt)"("Value"=w82) -> ()  [unwired: 2 in, 2 out]
      n44 = property on="FaktorMod0" class="Arr (strikt)"("Value"=w81) -> ()  [unwired: 2 in, 2 out]
      n45 = property on="FaktorMod1" class="Arr (strikt)"("Value"=w80) -> ()  [unwired: 2 in, 2 out]
      n46 = property on="FaktorMod2B" class="Arr (strikt)"("Value"=w78) -> ()  [unwired: 2 in, 2 out]
      n47 = property on="MWabfragenMod0" class="Arr (strikt)"("Value"=w77) -> ()  [unwired: 2 in, 2 out]
      n48 = property on="FaktorMod2A" class="Arr (strikt)"("Value"=w79) -> ()  [unwired: 2 in, 2 out]
      n49 = property on="MWabfragenMod1" class="Arr (strikt)"("Value"=w76) -> ()  [unwired: 2 in, 2 out]
      n50 = property on="MWabfragenMod2A" class="Arr (strikt)"("Value"=w75) -> ()  [unwired: 2 in, 2 out]
      n51 = property on="MWabfragenMod2B" class="Arr (strikt)"("Value"=w74) -> ()  [unwired: 2 in, 2 out]
      n52 = property on="Modul1/AI koeff" class="Arr (strikt)"("Value"=w73) -> ()  [unwired: 2 in, 2 out]
      n53 = property on="Modul3/AI koeff" class="Arr (strikt)"("Value"=w71) -> ()  [unwired: 2 in, 2 out]
      n54 = property on="Traps/MachsKoeff T(R)" class="Arr (strikt)"("Value"=w70) -> ()  [unwired: 2 in, 2 out]
      n55 = property on="Modul1/AIsNamen" class="Arr (strikt)"("Value"=w69) -> ()  [unwired: 2 in, 2 out]
      n56 = property on="Modul2/AIsNamen" class="Arr (strikt)"("Value"=w68) -> ()  [unwired: 2 in, 2 out]
      n57 = property on="Modul3/AIsNamen" class="Arr (strikt)"("Value"=w67) -> ()  [unwired: 2 in, 2 out]
      n58 = property on="Modul2/AI koeff" class="Arr (strikt)"("Value"=w72) -> ()  [unwired: 2 in, 2 out]
      n59 = property on="DIOsMod0Name" class="Arr (strikt)"("Value"=w66) -> ()  [unwired: 2 in, 2 out]
      n60 = property on="DIOsMod1Name" class="Arr (strikt)"("Value"=w65) -> ()  [unwired: 2 in, 2 out]
      n61 = property on="DIOsMod2AName" class="Arr (strikt)"("Value"=w64) -> ()  [unwired: 2 in, 2 out]
      n62 = property on="DIOsMod2BName" class="Arr (strikt)"("Value"=w63) -> ()  [unwired: 2 in, 2 out]
      n63 = property on="ReglerNameMod0" class="Arr (strikt)"("Value"=w62) -> ()  [unwired: 2 in, 2 out]
      n64 = property on="ReglerNameMod1" class="Arr (strikt)"("Value"=w61) -> ()  [unwired: 2 in, 2 out]
      n65 = property on="ReglerNameMod2A" class="Arr (strikt)"("Value"=w60) -> ()  [unwired: 2 in, 2 out]
      "Schnelle Heizungen" <- string[] ["Trap1 [°C]", "Trap2 [°C]", "PreCol1 [°C]", "PreCol2 [°C]", "MainCol1 [°C]", "MainCol2 [°C]"]
    }
    frame #1 {
      n66 = while {
        tunnel: ["DIOsMod0Name"] -> w119
        tunnel: ["DIOsMod1Name"] -> w118
        tunnel: ["DIOsMod2AName"] -> w117
        tunnel: ["DIOsMod2BName"] -> w116
        tunnel: ["ReglerNameMod0"] -> w115
        tunnel: ["ReglerNameMod1"] -> w114
        tunnel: ["ReglerNameMod2A"] -> w113
        tunnel: ["ReglerNameMod2B"] -> w112
        tunnel: [w138] -> w111
        tunnel: ["ReglerNameMod2B"] -> w110
        tunnel: ["ReglerNameMod2A"] -> w109
        tunnel: ["ReglerNameMod1"] -> w108
        tunnel: ["ReglerNameMod0"] -> w107
        tunnel: ["DIOsMod0Name"] -> w105
        tunnel: ["DIOsMod1Name"] -> w104
        tunnel: ["DIOsMod2AName"] -> w103
        tunnel: ["DIOsMod2BName"] -> w102
        tunnel: ["LangsameHeizungen"] -> w101
        tunnel: ["Metavariablen"] -> w99
        tunnel: ["Metavariablen"] -> w98
        stop <- "EinstellungenFertig" stop-if-true
        n67 = Wait (ms)(milliseconds to wait=u32 500 ("Zu wartende ms")) -> ()  [unwired: 1 out]
        n68 = case shown="True" "AIsNamenZurücksetzen" {
          frame False {
          }
          frame True {
            w204 = 32 ("Länge")
            w205 = string[] ["Mod1/AI0", "Mod1/AI1", "Mod1/AI2", "Mod1/AI3", "Mod1/AI4", "Mod1/AI5", "Mod1/AI6", "Mod1/AI7", "Mod1/AI8", "Mod1/AI9", "Mod1/AI10", "Mod1/AI11", "Mod1/AI12", "Mod1/AI13", "Mod1/AI14", "Mod1/AI15", "Mod1/AI16", "Mod1/AI17", "Mod1/AI18", "Mod1/AI19", "Mod1/AI20", "Mod1/AI21", "Mod1/AI22", "Mod1/AI23", "Mod1/AI24", "Mod1/AI25", "Mod1/AI26", "Mod1/AI27", "Mod1/AI28", "Mod1/AI29", "Mod1/AI30", "Mod1/AI31", "Mod2/AI0", "Mod2/AI1", "Mod2/AI2", "Mod2/AI3", "Mod2/AI4", "Mod2/AI5", "Mod2/AI6", "Mod2/AI7", "Mod2/AI8", "Mod2/AI9", "Mod2/AI10", "Mod2/AI11", "Mod2/AI12", "Mod2/AI13", "Mod2/AI14", "Mod2/AI15", "Mod2/AI16", "Mod2/AI17", "Mod2/AI18", "Mod2/AI19", "Mod2/AI20", "Mod2/AI21", "Mod2/AI22", "Mod2/AI23", "Mod2/AI24", "Mod2/AI25", "Mod2/AI26", "Mod2/AI27", "Mod2/AI28", "Mod2/AI29", "Mod2/AI30", "Mod2/AI31", "Mod3/AI0", "Mod3/AI1", "Mod3/AI2", "Mod3/AI3", "Mod3/AI4", "Mod3/AI5", "Mod3/AI6", "Mod3/AI7", "Mod3/AI8", "Mod3/AI9", "Mod3/AI10", "Mod3/AI11", "Mod3/AI12", "Mod3/AI13", "Mod3/AI14", "Mod3/AI15", "Mod3/AI16", "Mod3/AI17", "Mod3/AI18", "Mod3/AI19", "Mod3/AI20", "Mod3/AI21", "Mod3/AI22", "Mod3/AI23", "Mod3/AI24", "Mod3/AI25", "Mod3/AI26", "Mod3/AI27", "Mod3/AI28", "Mod3/AI29", "Mod3/AI30", "Mod3/AI31"] ("Array 2")
            n69 = Array Subset(array=w205, index=32 ("Index"), length=w204) -> (w201:string[])
            n70 = Array Subset(array=w205, index=0 ("Index"), length=w204) -> (w202:string[])
            n71 = Array Subset(array=w205, index=64 ("Index"), length=w204) -> (w200:string[])
            n72 = local write "Modul2/AIsNamen"(w201) -> ()
            n73 = local write "Modul1/AIsNamen"(w202) -> ()
            n74 = local write "Modul3/AIsNamen"(w200) -> ()
          }
        }
        n75 = Array Size(array="ReglerNameMod0") -> (size(s)=w188:i32)
        n76 = Array Size(array="ReglerNameMod1") -> (size(s)=w187:i32)
        n77 = Array Size(array="ReglerNameMod2A") -> (size(s)=w186:i32)
        n78 = Array Size(array="ReglerNameMod2B") -> (size(s)=w185:i32)
        n79 = Build Array "Anzahl Horst/Modul"(w188, w187, w186, w185) -> (w137:i32[])
        n80 = flat-sequence {
          tunnel: w137 -> [w198]
          tunnel: [w199] -> w136
          frame #0 {
            "AnzahlRegler/Modul" <- w198
          }
          frame #1 {
            n81 = local read "AnzahlRegler/Modul"() -> (w199:i32[])
          }
        }
        n82 = Build Array (concatenate)("Modul1/AIsNamen", "Modul2/AIsNamen", "Modul3/AIsNamen") -> (w138:string[])
        n83 = Bundle("DIOsMod0Nr"="DIOsMod0Nr", "DIOsMod1Nr"="DIOsMod1Nr", "DIOsMod2ANr"="DIOsMod2ANr", "DIOsMod2BNr"="DIOsMod2BNr", "AIsLH"="AIsLH", "AnzahlRegler/Modul"=w136, "Regler für den Probenfluß"="Regler für den Probenfluß", "SPvorgebenMod0"="SPvorgebenMod0", "SPvorgebenMod1"="SPvorgebenMod1", "SPvorgebenMod2A"="SPvorgebenMod2A", "SPvorgebenMod2B"="SPvorgebenMod2B", "MWAntwortMod0"="MWAntwortMod0", "MWAntwortMod1"="MWAntwortMod1", "MWAntwortMod2A"="MWAntwortMod2A", "MWAntwortMod2B"="MWAntwortMod2B", "FaktorMod0"="FaktorMod0", "FaktorMod1"="FaktorMod1", "FaktorMod2A"="FaktorMod2A", "FaktorMod2B"="FaktorMod2B", "MWabfragenMod0"="MWabfragenMod0", "MWabfragenMod1"="MWabfragenMod1", "MWabfragenMod2A"="MWabfragenMod2A", "MWabfragenMod2B"="MWabfragenMod2B", "Modul1/AI koeff"="Modul1/AI koeff", "Modul2/AI koeff"="Modul2/AI koeff", "Modul3/AI koeff"="Modul3/AI koeff", "Traps/MachsKoeff T(R)"="Traps/MachsKoeff T(R)", "Modul1/AIsNamen"="Modul1/AIsNamen", "Modul2/AIsNamen"="Modul2/AIsNamen", "Modul3/AIsNamen"="Modul3/AIsNamen", "DIOsMod0Name"="DIOsMod0Name", "DIOsMod1Name"="DIOsMod1Name", "DIOsMod2AName"="DIOsMod2AName", "DIOsMod2BName"="DIOsMod2BName", "ReglerNameMod0"="ReglerNameMod0", "ReglerNameMod1"="ReglerNameMod1", "ReglerNameMod2A"="ReglerNameMod2A", "ReglerNameMod2B"="ReglerNameMod2B", "Startmethode"="Startmethode", "Dateiordner Housekeeping"="Dateiordner Housekeeping", "Dateiname Housekeeping"="Dateiname Housekeeping", "DateiordnerECD1"="DateiordnerECD1", "DateinameECD1"="DateinameECD1", "DateiordnerECD2"="DateiordnerECD2", "DateinameECD2"="DateinameECD2", "LangsameHeizungen"="LangsameHeizungen", "ModuleLH"="ModuleLH", "Metavariablen"="Metavariablen", "Modul1/AI sicherer Bereich"="Modul1/AI sicherer Bereich", "Modul2/AI sicherer Bereich"="Modul2/AI sicherer Bereich", "Modul3/AI sicherer Bereich"="Modul3/AI sicherer Bereich", "Traps/Machs sicherer Bereich"="Traps/Machs sicherer Bereich", "ReglerMod0 sicherer Bereich"="ReglerMod0 sicherer Bereich", "ReglerMod1 sicherer Bereich"="ReglerMod1 sicherer Bereich", "ReglerMod2A sicherer Bereich"="ReglerMod2A sicherer Bereich", "ReglerMod2B sicherer Bereich"="ReglerMod2B sicherer Bereich", "Metavariablen grüner Bereich"="Metavariablen grüner Bereich", "Traps/MachsKoeff R(U)"="Traps/MachsKoeff R(U)", "LHGruppe"="LHGruppe") -> (w133:T5)  [unwired: 1 in]
        n84 = case shown="True" "EinstellungenSpeichern" {
          tunnel: w133 -> [_ w194]
          frame False {
          }
          frame True {
            n85 = Open/Create/Replace File(file path (use dialog)=path "c:/einstellungen.pery" ("Dateipfad Einstellungen"), operation (0:open)=T6."replace or create" ("Operation (0:Öffnen)")) -> (refnum out=w196:refnum<file>, error out=w193:errorcluster)  [unwired: 4 in, 1 out]
            n86 = Write to Binary File(file (use dialog)=w196, data=w194, error in=w193) -> (refnum out=w195:refnum<file>, error out=w192:errorcluster)  [unwired: 3 in, 1 out]
            n87 = Close File(refnum=w195, error in=w192) -> (error out=w191:errorcluster)  [unwired: 1 out]
            n88 = call <vilib>:"Simple Error Handler.vi"("error in (no error)"=w191) -> ()  [unwired: 4 in, 5 out]
          }
        }
      }
      n89 = Build Array (concatenate)(w107, w108, w109, w110) -> (w106:string[])
    }
    frame #2 {
      w221 = string[] ["<", "<=", "=", ">=", ">", "=/="] ("Strings []")
      n90 = for {
        tunnel: w216 -> [w241] mode=indexing
        tunnel: [w239] -> w215 mode=indexing
        n91 = Concatenate Strings(w241, " heizen?" ("String")) -> (w239:string)
      }
      n92 = Build Array (concatenate)(w228, w227, w226, w225) -> (w209:string[])
      n93 = Build Array (concatenate)(w209, string[] ["Heizen?Trap1", "Heizen?Trap2", "Heizen?PreMach1", "Heizen?PreMach2", "Heizen?MainMach1", "Heizen?MainMach2", "Methodennummer", "STOPP!!!"], w215, w217, "PositionMPV", w212) -> (w223:string[])
      n94 = Build Array (concatenate)(w230, string[] ["T-Trap1", "T-Trap2", "T-PreMach1", "T-PreMach2", "T-MainMach1", "T-MainMach2"], w217, string[] ["Gesamte Zeit", "Methodenzeit", "Zykluszeit Mod0", "Zykluszeit Mod1", "Zykluszeit Mod2A", "Zykluszeit Mod2B"] ("Array"), "PositionMPV", w214) -> (w222:string[])
      n95 = property on="Vergleichsoperator2" class="Ring (strikt)"("Strings []"=w221) -> ()  [unwired: 2 in, 2 out]
      n96 = while {
        tunnel: w238 -> [w310]
        tunnel: w237 -> [w309]
        tunnel: w236 -> [w308]
        tunnel: w235 -> [w307]
        tunnel: w234 -> [w306]
        tunnel: w233 -> [w305]
        tunnel: w232 -> [w304]
        tunnel: w231 -> [w303]
        shift-right: [w263] -> w210
        shift-left: w208 -> [w245]
        tunnel: w222 -> [w270]
        tunnel: w221 -> [w269]
        tunnel: w223 -> [w268]
        tunnel: w219 -> [w262]
        stop <- w300 stop-if-true
        n97 = Index Array(array=w245, index="Methode Nummer") -> (element=w299:T7)
        n98 = Unbundle(w299) -> ("Zykluslängen [s]"=w298:dbl[], "ZeitpktDIOsMod0"=w297:dbl[], "ZeitpktDIOsMod1"=w296:dbl[], "ZeitpktDIOsMod2A"=w295:dbl[], "ZeitpktDIOsMod2B"=w294:dbl[], "DIOsSPMod0"=w293:bool[][], "DIOsSPMod1"=w292:bool[][], "DIOsSPMod2A"=w291:bool[][], "DIOsSPMod2B"=w290:bool[][], "Mod0HorstZeitpkt"=w289:dbl[], "Mod1HorstZeitpkt"=w288:dbl[], "Mod2AHorstZeitpkt"=w287:dbl[], "Mod2BHorstZeitpkt"=w286:dbl[], "HorstSPMod0"=w285:dbl[][], "HorstSPMod1"=w284:dbl[][], "HorstSPMod2A"=w283:dbl[][], "HorstSPMod2B"=w282:dbl[][], "LHSetpoints"=w281:dbl[], "LHHeizen?"=w280:bool[], "ZPktFPGABoolesch"=w279:dbl[], "FPGABoolesch"=w278:bool[][], "ZeitpktFPGAPID"=w277:dbl[], "FPGAPID"=w242:T4, "ZeitpktFPGAFixp"=w276:dbl[], "SHSetpoints"=w275:dbl[][], "t_PreMach1"=w274:dbl[], "T_PreMach1"=w273:dbl[], "t_PreMach2"=w272:dbl[], "T_PreMach2"=w271:dbl[], "PIDs für \"träge\" Heizungen"=w267:T8, "Zwangsbedingungen"=w266:dbl[][], "Dateien fürs MS schicken?"=w265:bool, "ZeitpunkteMPV"=w258:dbl[], "SPMPV"=w257:i32[], "ZeitpktMS-1"=w260:dbl, "ZeitpktMS-2"=w259:dbl, "Int.Start1"=w256:dbl, "Int.Stop1"=w255:dbl, "Int.Start2"=w254:dbl, "Int.Stop2"=w253:dbl, "Methodenname"=w261:string, "t_MainMach1"=w252:dbl[], "T_MainMach1"=w251:dbl[], "t_MainMach2"=w250:dbl[], "T_MainMach2"=w249:dbl[])
        n99 = property on="LHHeizen?" class="Arr (strikt)"("Value"=w280) -> ()  [unwired: 2 in, 2 out]
        n100 = property on="FPGAPID" class="Arr (strikt)"("Value"=w242) -> ()  [unwired: 2 in, 2 out]
        n101 = property on="SPMPV" class="Arr (strikt)"("Value"=w257) -> ()  [unwired: 2 in, 2 out]
        n102 = property on="Int.Start1" class="DigWert (strikt)"("Value"=w256) -> ()  [unwired: 2 in, 2 out]
        n103 = property on="Int.Stop1" class="DigWert (strikt)"("Value"=w255) -> ()  [unwired: 2 in, 2 out]
        n104 = property on="Int.Start2" class="DigWert (strikt)"("Value"=w254) -> ()  [unwired: 2 in, 2 out]
        n105 = property on="Int.Stop2" class="DigWert (strikt)"("Value"=w253) -> ()  [unwired: 2 in, 2 out]
        n106 = property on="T_MainMach2" class="Arr (strikt)"("Value"=w249) -> ()  [unwired: 2 in, 2 out]
        n107 = property on="Zykluslängen [s]" class="Arr (strikt)"("Value"=w298) -> ()  [unwired: 2 in, 2 out]
        n108 = property on="ZeitpktDIOsMod0" class="Arr (strikt)"("Value"=w297) -> ()  [unwired: 2 in, 2 out]
        n109 = property on="Mod2BHorstZeitpkt" class="Arr (strikt)"("Value"=w286) -> ()  [unwired: 2 in, 2 out]
        n110 = property on="HorstSPMod0" class="Arr (strikt)"("Value"=w285) -> ()  [unwired: 2 in, 2 out]
        n111 = property on="LHSetpoints" class="Arr (strikt)"("Value"=w281) -> ()  [unwired: 2 in, 2 out]
        n112 = property on="ZPktFPGABoolesch" class="Arr (strikt)"("Value"=w279) -> ()  [unwired: 2 in, 2 out]
        n113 = property on="FPGABoolesch" class="Arr (strikt)"("Value"=w278) -> ()  [unwired: 2 in, 2 out]
        n114 = property on="T_PreMach2" class="Arr (strikt)"("Value"=w271) -> ()  [unwired: 2 in, 2 out]
        n115 = property on="PIDs für \"träge\" Heizungen" class="Arr (strikt)"("Value"=w267) -> ()  [unwired: 2 in, 2 out]
        n116 = while {
          tunnel: w309 -> [w418]
          tunnel: w308 -> [w417]
          tunnel: w307 -> [w416]
          tunnel: w306 -> [w415]
          tunnel: w305 -> [w414]
          tunnel: w303 -> [w413]
          tunnel: w304 -> [w412]
          tunnel: w310 -> [w382]
          tunnel: [w381] -> w301
          tunnel: [w344] -> w302
          tunnel: ["EditorBeenden"] -> w300
          tunnel: w270 -> [w367]
          shift-right: [w362] -> _
          shift-left: w266 -> [w366]
          tunnel: w269 -> [w365]
          tunnel: w268 -> [w364]
          tunnel: ["AllesSpeichern"] -> w264
          tunnel: ["MethodeDuplizieren"] -> w247
          stop <- w336 stop-if-true
          n117 = for {
            tunnel: w366 -> [w427] mode=indexing
            tunnel: w367 -> [w423]
            tunnel: w365 -> [w422]
            tunnel: w364 -> [w441]
            tunnel: [w435] -> w375 mode=indexing
            n118 = Index Array(array=w427, index=0 ("Index")) -> (element=w447:dbl)
            n119 = Index Array(array=w427, index=1 ("Index")) -> (element=w445:dbl)
            n120 = Index Array(array=w427, index=3 ("Index")) -> (element=w429:dbl)
            n121 = Index Array(array=w427, index=4 ("Index")) -> (element=w428:dbl)
            n122 = Index Array(array=w427, index=6 ("Index")) -> (element=w443:dbl)
            n123 = To Long Integer(number=w447) -> (32bit integer=w446:i32)
            n124 = To Long Integer(number=w445) -> (32bit integer=w444:i32)
            n125 = To Long Integer(number=w429) -> (32bit integer=w426:i32)
            n126 = To Long Integer(number=w428) -> (32bit integer=w425:i32)
            n127 = To Long Integer(number=w443) -> (32bit integer=w442:i32)
            n128 = Index Array(array=w427, index=2 ("Index")) -> (element=w440:dbl)
            n129 = Index Array(array=w427, index=5 ("Index")) -> (element=w424:dbl)
            n130 = Index Array(array=w427, index=7 ("Index")) -> (element=w439:dbl)
            n131 = Index Array(array=w423, index=w446) -> (element=w438:string)
            n132 = Index Array(array=w422, index=w444) -> (element=w437:string)
            n133 = Index Array(array=w423, index=w426) -> (element=w421:string)
            n134 = Index Array(array=w422, index=w425) -> (element=w420:string)
            n135 = Index Array(array=w441, index=w442) -> (element=w433:string)
            n136 = Number To Exponential String(number=w440) -> (E-format string=w436:string)  [unwired: 3 in]
            n137 = Number To Exponential String(number=w424) -> (E-format string=w419:string)  [unwired: 3 in]
            n138 = Number To Exponential String(number=w439) -> (E-format string=w434:string)  [unwired: 3 in]
            n139 = Build Array(w438, w437, w436, w421, w420, w419, w433, w434) -> (w435:string[])
          }
          "ZwangsBedingungen" <- w375
          n140 = Wait (ms)(milliseconds to wait=u32 500 ("Zu wartende ms")) -> ()  [unwired: 1 out]
          n141 = Build Array("AbfragbareVariablen1", "Vergleichsoperator1", "Wert1", "AbfragbareVariablen2", "Vergleichsoperator2", "Wert2", "BedienbareVariablen", "Ausgangswert") -> (w372:dbl[])
          n142 = case shown="False" "Bedingung übernehmen" {
            tunnel: w366 -> [w457 w460]
            tunnel: w372 -> [_ w459]
            tunnel: [w457 w458] -> w373
            frame False {
            }
            frame True {
              n143 = Build Array (concatenate)(w460, w459) -> (w458:dbl[][])
            }
          }
          n144 = case shown="True" "löschen" {
            tunnel: w373 -> [w453 w456]
            tunnel: [w453 w454] -> w362
            frame False {
            }
            frame True {
              n145 = Delete From Array(array=w456, index (row)="Bedingung Nr. X") -> (array with subset deleted=w454:dbl[][])  [unwired: 2 in, 1 out]
            }
          }
          n146 = Or(x="MethodeSpeichern", y="EditorBeenden") -> (x .or. y?=w379:bool)
          n147 = Or(x=w379, y="MethodeLaden") -> (x .or. y?=w346:bool)
          n148 = local write "Zwangsbedingungen"(w362) -> ()
          n149 = Or(x=w346, y="AllesSpeichern") -> (x .or. y?=w337:bool)
          n150 = Or(x="MethodeDuplizieren", y=w337) -> (x .or. y?=w336:bool)
          n151 = Or(x="AllesSpeichern", y="MethodeSpeichern") -> (x .or. y?=w344:bool)
          n152 = Bundle("Zykluslängen [s]"="Zykluslängen [s]", "ZeitpktDIOsMod0"="ZeitpktDIOsMod0", "ZeitpktDIOsMod1"="ZeitpktDIOsMod1", "ZeitpktDIOsMod2A"="ZeitpktDIOsMod2A", "ZeitpktDIOsMod2B"="ZeitpktDIOsMod2B", "DIOsSPMod0"="DIOsSPMod0", "DIOsSPMod1"="DIOsSPMod1", "DIOsSPMod2A"="DIOsSPMod2A", "DIOsSPMod2B"="DIOsSPMod2B", "Mod0HorstZeitpkt"="Mod0HorstZeitpkt", "Mod1HorstZeitpkt"="Mod1HorstZeitpkt", "Mod2AHorstZeitpkt"="Mod2AHorstZeitpkt", "Mod2BHorstZeitpkt"="Mod2BHorstZeitpkt", "HorstSPMod0"="HorstSPMod0", "HorstSPMod1"="HorstSPMod1", "HorstSPMod2A"="HorstSPMod2A", "HorstSPMod2B"="HorstSPMod2B", "LHSetpoints"="LHSetpoints", "LHHeizen?"="LHHeizen?", "ZPktFPGABoolesch"="ZPktFPGABoolesch", "FPGABoolesch"="FPGABoolesch", "ZeitpktFPGAPID"="ZeitpktFPGAPID", "FPGAPID"="FPGAPID", "ZeitpktFPGAFixp"="ZeitpktFPGAFixp", "SHSetpoints"="SHSetpoints", "t_PreMach1"="t_PreMach1", "T_PreMach1"="T_PreMach1", "t_PreMach2"="t_PreMach2", "T_PreMach2"="T_PreMach2", "PIDs für \"träge\" Heizungen"="PIDs für \"träge\" Heizungen", "Zwangsbedingungen"="Zwangsbedingungen", "Dateien fürs MS schicken?"="Dateien fürs MS schicken?", "ZeitpunkteMPV"="ZeitpunkteMPV", "SPMPV"="SPMPV", "ZeitpktMS-1"="ZeitpktMS-1", "ZeitpktMS-2"="ZeitpktMS-2", "Int.Start1"="Int.Start1", "Int.Stop1"="Int.Stop1", "Int.Start2"="Int.Start2", "Int.Stop2"="Int.Stop2", "Methodenname"="Methodenname", "t_MainMach1"="t_MainMach1", "T_MainMach1"="T_MainMach1", "t_MainMach2"="t_MainMach2", "T_MainMach2"="T_MainMach2") -> (w381:T9)  [unwired: 1 in]
          "DIOsMod0Name" <- w382
          "DIOsMod1Name" <- w418
          "DIOsMod2AName" <- w417
          "DIOsMod2BName" <- w416
          "HorstMod0Name" <- w415
          "HorstMod2BName" <- w412
          "HorstMod2AName" <- w413
          "HorstMod1Name" <- w414
        }
        n153 = property on="DIOsSPMod1" class="Arr (strikt)"("Value"=w292) -> ()  [unwired: 2 in, 2 out]
        n154 = property on="DIOsSPMod2A" class="Arr (strikt)"("Value"=w291) -> ()  [unwired: 2 in, 2 out]
        n155 = property on="HorstSPMod1" class="Arr (strikt)"("Value"=w284) -> ()  [unwired: 2 in, 2 out]
        n156 = property on="HorstSPMod2A" class="Arr (strikt)"("Value"=w283) -> ()  [unwired: 2 in, 2 out]
        n157 = property on="HorstSPMod2B" class="Arr (strikt)"("Value"=w282) -> ()  [unwired: 2 in, 2 out]
        n158 = property on="ZeitpktFPGAPID" class="Arr (strikt)"("Value"=w277) -> ()  [unwired: 2 in, 2 out]
        n159 = property on="ZeitpktFPGAFixp" class="Arr (strikt)"("Value"=w276) -> ()  [unwired: 2 in, 2 out]
        n160 = property on="SHSetpoints" class="Arr (strikt)"("Value"=w275) -> ()  [unwired: 2 in, 2 out]
        n161 = property on="t_PreMach1" class="Arr (strikt)"("Value"=w274) -> ()  [unwired: 2 in, 2 out]
        n162 = property on="T_PreMach1" class="Arr (strikt)"("Value"=w273) -> ()  [unwired: 2 in, 2 out]
        n163 = property on="t_PreMach2" class="Arr (strikt)"("Value"=w272) -> ()  [unwired: 2 in, 2 out]
        n164 = property on="ZeitpktDIOsMod1" class="Arr (strikt)"("Value"=w296) -> ()  [unwired: 2 in, 2 out]
        n165 = property on="ZeitpktDIOsMod2A" class="Arr (strikt)"("Value"=w295) -> ()  [unwired: 2 in, 2 out]
        n166 = property on="ZeitpktDIOsMod2B" class="Arr (strikt)"("Value"=w294) -> ()  [unwired: 2 in, 2 out]
        n167 = property on="DIOsSPMod0" class="Arr (strikt)"("Value"=w293) -> ()  [unwired: 2 in, 2 out]
        n168 = property on="DIOsSPMod2B" class="Arr (strikt)"("Value"=w290) -> ()  [unwired: 2 in, 2 out]
        n169 = property on="Mod0HorstZeitpkt" class="Arr (strikt)"("Value"=w289) -> ()  [unwired: 2 in, 2 out]
        n170 = property on="Mod1HorstZeitpkt" class="Arr (strikt)"("Value"=w288) -> ()  [unwired: 2 in, 2 out]
        n171 = property on="Mod2AHorstZeitpkt" class="Arr (strikt)"("Value"=w287) -> ()  [unwired: 2 in, 2 out]
        n172 = property on="Dateien fürs MS schicken?" class="Bool. (strikt)"("Value"=w265) -> ()  [unwired: 2 in, 2 out]
        n173 = property on="ZeitpunkteMPV" class="Arr (strikt)"("Value"=w258) -> ()  [unwired: 2 in, 2 out]
        n174 = property on="ZeitpktMS-1" class="DigWert (strikt)"("Value"=w260) -> ()  [unwired: 2 in, 2 out]
        n175 = property on="ZeitpktMS-2" class="DigWert (strikt)"("Value"=w259) -> ()  [unwired: 2 in, 2 out]
        n176 = property on="Methodenname" class="Str"("Value"=w261) -> ()  [unwired: 2 in, 2 out]
        n177 = property on="t_MainMach1" class="Arr (strikt)"("Value"=w252) -> ()  [unwired: 2 in, 2 out]
        n178 = property on="T_MainMach1" class="Arr (strikt)"("Value"=w251) -> ()  [unwired: 2 in, 2 out]
        n179 = property on="t_MainMach2" class="Arr (strikt)"("Value"=w250) -> ()  [unwired: 2 in, 2 out]
        n180 = case shown="True" "MethodeLöschen" {
          tunnel: w245 -> [w311 w315]
          tunnel: [w311 w312] -> w244
          tunnel: "Methode Nummer" -> [_ w313]
          frame False {
          }
          frame True {
            n181 = invoke on="MethodeLöschen" class="Bool (strict)" method="Std wiederherstellen"() -> ()  [unwired: 3 in, 3 out]
            n182 = Delete From Array(array=w315, length=1, index=w313) -> (array with subset deleted=w312:T1)  [unwired: 1 out]
          }
        }
        n183 = case shown="True" w247 {
          tunnel: w244 -> [w316 w319]
          tunnel: [w316 w318] -> w248
          tunnel: "Methode Nummer" -> [_ w320]
          frame False {
          }
          frame True {
            n184 = Index Array(array=w319, index=w320) -> (element=w317:T7)
            n185 = Build Array (concatenate)(w319, w317) -> (w318:T1)
          }
        }
        n186 = case shown="True" w302 {
          tunnel: w248 -> [w329 w335]
          tunnel: w301 -> [_ w330]
          tunnel: [w329 w331] -> w263
          tunnel: "Methode Nummer" -> [_ w332]
          frame False {
          }
          frame True {
            n187 = Delete From Array(array=w335, length=1 ("Länge"), index=w332) -> (array with subset deleted=w333:T1)  [unwired: 1 out]
            n188 = Insert Into Array(array=w333, index=w332, new element=w330) -> (w331:T1)
          }
        }
        n189 = case shown="True" w264 {
          tunnel: w263 -> [_ w326]
          tunnel: w262 -> [_ w321]
          frame False {
          }
          frame True {
            n190 = Open/Create/Replace File(file path (use dialog)=w321, operation (0:open)=T6."replace or create" ("Operation (0:Öffnen)")) -> (refnum out=w325:refnum<file>, error out=w327:errorcluster)  [unwired: 4 in, 1 out]
            n191 = Write to Binary File(file (use dialog)=w325, data=w326, error in=w327) -> (refnum out=w323:refnum<file>, error out=w324:errorcluster)  [unwired: 3 in, 1 out]
            n192 = Close File(refnum=w323, error in=w324) -> (error out=w322:errorcluster)  [unwired: 1 out]
            n193 = call <vilib>:"Simple Error Handler.vi"("error in (no error)"=w322) -> ()  [unwired: 4 in, 5 out]
          }
        }
      }
      "Methoden" <- w210
      n194 = property on="BedienbareVariablen" class="Ring (strikt)"("Strings []"=w223) -> ()  [unwired: 2 in, 2 out]
      n195 = property on="AbfragbareVariablen1" class="Ring (strikt)"("Strings []"=w222) -> ()  [unwired: 2 in, 2 out]
      n196 = property on="AbfragbareVariablen2" class="Ring (strikt)"("Strings []"=w222) -> ()  [unwired: 2 in, 2 out]
      n197 = property on="Vergleichsoperator1" class="Ring (strikt)"("Strings []"=w221) -> ()  [unwired: 2 in, 2 out]
      "LangsameHeizungen" <- w220
    }
  }
  n198 = call <vilib>:"Simple Error Handler.vi"("error in (no error)"=w16) -> ()  [unwired: 4 in, 5 out]
  n199 = Open/Create/Replace File(file path (use dialog)=path "C:/methoden.pery" ("Dateipfad Methoden")) -> (refnum out=w14:refnum<file>, error out=w13:errorcluster)  [unwired: 5 in, 1 out]
  n200 = Read from Binary File(5:T1 [] ("Methoden 2"), 8:w13, 11:w14) -> (0:w11:errorcluster, 2:w4:T1, 3:w12:refnum<file>)  [unwired: 3 in, 1 out]
  n201 = Close File(refnum=w12, error in=w11) -> (path=w3:path, error out=w10:errorcluster)
  n202 = call <vilib>:"Simple Error Handler.vi"("error in (no error)"=w10) -> ()  [unwired: 4 in, 5 out]
